vi "Autonomous Independent.vi"   [LabVIEW 2015]
doc: "This VI is called when autonomous begins, and will automatically be terminated when autonomous ends. You can carry out timed or sensor driven robot movement independently without needing to return to the caller."
uses:
  <vilib>/Rock Robotics/WPI/Utilities/WPI_GetSetVariantRefNum.vi
  <vilib>/Rock Robotics/Network Tables/NT Read String.vi
  <vilib>/Rock Robotics/Network Tables/NT Write Numeric Array.vi
  <vilib>/Rock Robotics/WPI/RobotDrive/WPI_RobotDriveArcadeDrive_Standard(NoSaturation).vi
  Robot Global Data.vi
panel:
  # "Be sure to right-click and choose Data Operations>>Make Current Value default if you want to save the array values with the VI"
types:
  T1 = typedef "WPI_JoystickDevRef.ctl" = cluster{"Device":T2}
  T2 = typedef "WPI_JoystickDeviceEnum.ctl" = enum16{"USB 0", "USB 1", "USB 2", "USB 3", "USB 4", "USB 5"}
  T3 = typedef "WPI_RobotDriveDevRef.ctl" = cluster{"DevStatus":errorcluster, "Motors[]":T4[], "Square Inputs":bool, "Max Output":dbl}
  T4 = typedef "WPI_MotorControlDeviceRef.ctl" = cluster{"DeviceStatus":errorcluster, "Type":T5, "PWM":cluster{"PWM Channel":T6, "DeadBand":T7}, "CAN":cluster{"Device Number":u8, "Control Mode":T8, "Semaphore":T9, "Max Vout":dbl, "TalonSRX Control Mode":T10}, "Invert":bool}
  T5 = typedef "WPI_MotorControlType.ctl" = enum16{"PWM", "CAN", "CANTalonSRX"}
  T6 = typedef "FPGA_DIOPWMChannel.ctl" = enum8{"PWM 0", "PWM 1", "PWM 2", "PWM 3", "PWM 4", "PWM 5", "PWM 6", "PWM 7", "PWM 8", "PWM 9", "PWM MXP 0", "PWM MXP 1", "PWM MXP 2", "PWM MXP 3", "PWM MXP 4", "PWM MXP 5", "PWM MXP 6", "PWM MXP 7", "PWM MXP 8", "PWM MXP 9", "Invalid"}
  T7 = typedef "WPI_PWMDeadband.ctl" = cluster{"Name":string, "maxPositivePwm":i32, "minPositivePwm":i32, "centerPwm":i32, "maxNegativePwm":i32, "minNegativePwm":i32, "angularRange":u16}
  T8 = typedef "WPI_CANJaguar_ControlMode.ctl" = enum8{"Percent VBus", "Current", "Speed", "Position", "Voltage"}
  T9 = typedef "Semaphore RefNum" = refnum<k1>
  T10 = typedef "WPI_CANTalonSRX_APIControlMode.ctl" = enum8{"Percent VBus", "Speed", "Position", "Slave", "Unchanged / Invalid", "Voltage Compensation", "Current", "Motion Profile"}
  T11 = typedef "WPI_AnalogChannelDevRef.ctl" = cluster{"DevStatus":errorcluster, "Analog Channel":T12}
  T12 = typedef "FPGA_AIChannel.ctl" = enum8{"AI 0", "AI 1", "AI 2", "AI 3", "AI MXP 0", "AI MXP 1", "AI MXP 2", "AI MXP 3", "Invalid"}
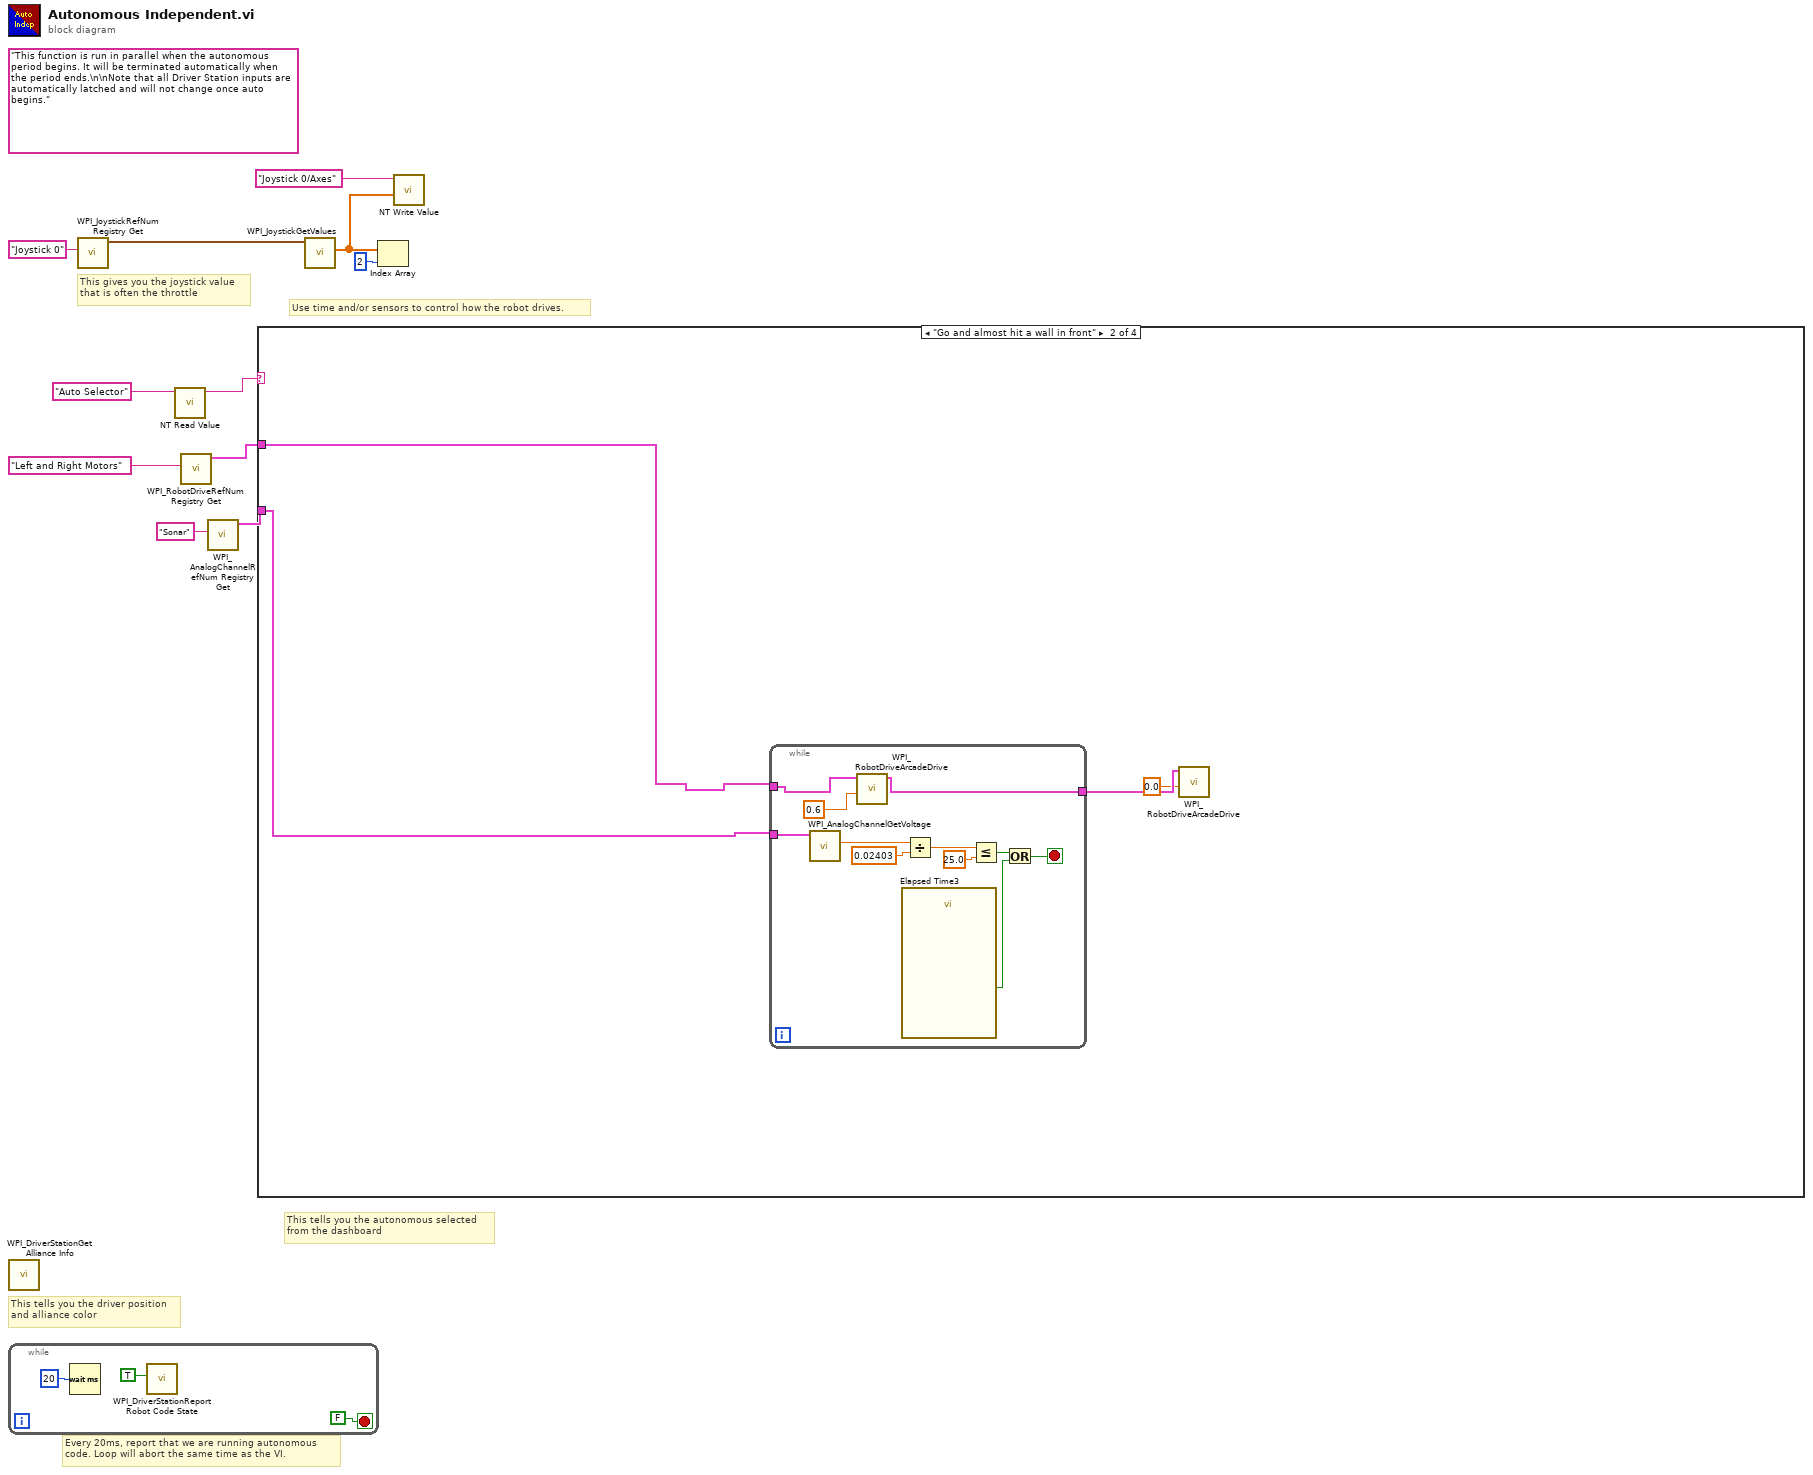
[diagram p0: block diagram]
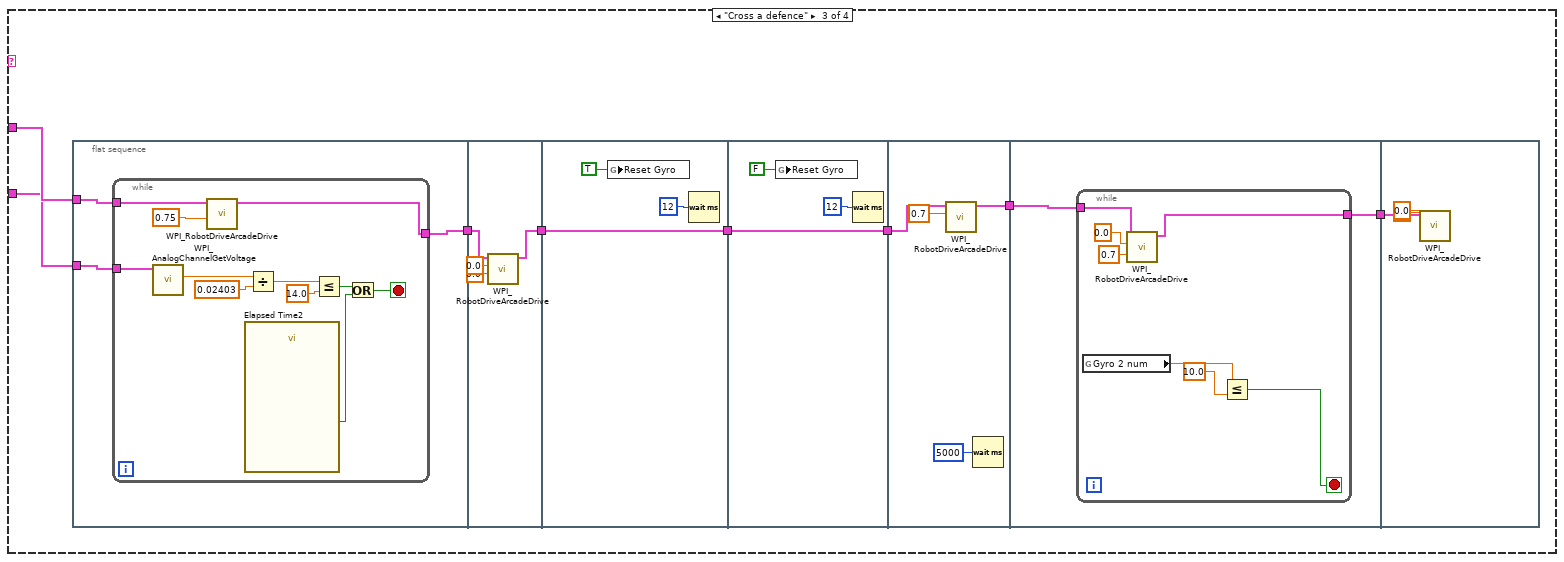
[diagram p3: hidden frame]
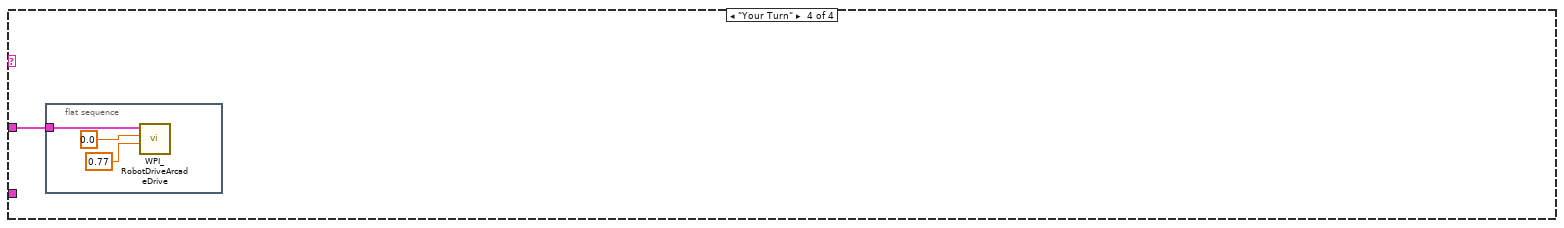
[diagram p4: hidden frame]
diagram:
  (unwired) "This function is run in parallel when the autonomous period begins. It will be terminated automatically when the period ends.\n\nNote that all Driver Station inputs are automatically latched and will not change once auto begins."
  # "This tells you the autonomous selected\nfrom the dashboard"
  # "Every 20ms, report that we are running autonomous\ncode. Loop will abort the same time as the VI."
  # "This gives you the joystick value\nthat is often the throttle"
  # "Use time and/or sensors to control how the robot drives."
  # "This tells you the driver position\nand alliance color"
  n1 = call <vilib>:"WPI_DriverStationGet Alliance Info.vi"() -> ()  [unwired: 12 out]
  n2 = while {
    stop <- FALSE stop-if-true
    n3 = Wait (ms)(milliseconds to wait=u32 20) -> ()  [unwired: 1 out]
    n4 = call <vilib>:"WPI_DriverStationReport Robot Code State.vi"("Autonomous"=TRUE) -> ()  [unwired: 10 in, 1 out]
  }
  n5 = call <vilib>:"WPI_JoystickRefNum Registry Get.vi"("refnum name"="Joystick 0") -> ("JoystickDevRef"=w10:T1)  [unwired: 1 in, 9 out]
  n6 = call-poly <vilib>:"NT Read Value.vi"("Name"="Auto Selector") -> ("String"=w7:string)  [unwired: 9 in, 1 out]
  n7 = call <vilib>:"WPI_RobotDriveRefNum Registry Get.vi"("refnum name"="Left and Right Motors") -> ("RobotDriveDevRef"=w3:T3)  [unwired: 9 in, 1 out]
  n8 = call <vilib>:"WPI_AnalogChannelRefNum Registry Get.vi"("refnum name"="Sonar") -> ("AIDeviceRef"=w1:T11)  [unwired: 9 in, 1 out]
  n9 = case shown="\"Go and almost hit a wall in front\"" w7 {
    tunnel: w1 -> [_ w18 w36 _]
    tunnel: w3 -> [_ w15 w37 w78]
    frame Default {
      # "You can put your main auto here, or you can right-click on the case and make any\nother frame be the default case."
      # "This is the frame that will execute if no selection is made, or if it is not recognized"
    }
    frame "Go and almost hit a wall in front" {
      n10 = while {
        tunnel: w18 -> [w28]
        tunnel: w15 -> [w20]
        tunnel: [w19] -> w17
        stop <- w23 stop-if-true
        n11 = call <vilib>:"WPI_AnalogChannelGetVoltage.vi"("AIDeviceRef"=w28) -> ("Voltage"=w27:dbl)  [unwired: 8 in, 2 out]
        n12 = call-poly <vilib>:"WPI_RobotDriveArcadeDrive.vi"("Y axis value"=0.6, "RobotDriveDevRef"=w20) -> ("RobotDriveDevRef"=w19:T3)  [unwired: 7 in, 2 out]
        n13 = call "Elapsed Time3"() -> ("Time has Elapsed"=w22:bool)  [unwired: 12 in, 7 out]
        n14 = Divide(x=w27, y=0.02403) -> (x/y=w25:dbl)
        n15 = Less Or Equal?(x=w25, y=25.0) -> (x <= y?=w24:bool)
        n16 = Or(x=w24, y=w22) -> (x .or. y?=w23:bool)
      }
      n17 = call-poly <vilib>:"WPI_RobotDriveArcadeDrive.vi"("Y axis value"=0.0, "RobotDriveDevRef"=w17) -> ()  [unwired: 7 in, 3 out]
    }
    frame "Cross a defence" {
      n18 = flat-sequence {
        tunnel: w37 -> [w40]
        tunnel: w36 -> [w39]
        tunnel: [w38] -> w31
        tunnel: w31 -> [w55]
        tunnel: [w54] -> w30
        tunnel: [w56] -> w34
        tunnel: w30 -> [w56]
        tunnel: [w59] -> w35
        tunnel: w34 -> [w59]
        tunnel: w35 -> [w65]
        tunnel: [w62] -> w33
        tunnel: w33 -> [w67]
        tunnel: [w66] -> w32
        tunnel: w32 -> [w77]
        frame #0 {
          n19 = while {
            tunnel: w39 -> [w49]
            tunnel: w40 -> [w51]
            tunnel: [w41] -> w38
            stop <- w43 stop-if-true
            n20 = call <vilib>:"WPI_AnalogChannelGetVoltage.vi"("AIDeviceRef"=w49) -> ("Voltage"=w48:dbl)  [unwired: 8 in, 2 out]
            n21 = call-poly <vilib>:"WPI_RobotDriveArcadeDrive.vi"("Y axis value"=0.75 ("X axis value"), "RobotDriveDevRef"=w51) -> ("RobotDriveDevRef"=w41:T3)  [unwired: 7 in, 2 out]
            n22 = call "Elapsed Time2"() -> ("Time has Elapsed"=w42:bool)  [unwired: 12 in, 7 out]
            n23 = Divide(x=w48, y=0.02403) -> (x/y=w46:dbl)
            n24 = Less Or Equal?(x=w46, y=14.0) -> (x <= y?=w44:bool)
            n25 = Or(x=w44, y=w42) -> (x .or. y?=w43:bool)
          }
        }
        frame #1 {
          n26 = call-poly <vilib>:"WPI_RobotDriveArcadeDrive.vi"("Y axis value"=0.0, "X axis value"=0.0, "RobotDriveDevRef"=w55) -> ("RobotDriveDevRef"=w54:T3)  [unwired: 6 in, 2 out]
        }
        frame #2 {
          n27 = global write "Robot Global Data.vi" "Reset Gyro"(TRUE) -> ()
          n28 = Wait (ms)(milliseconds to wait=u32 12) -> ()  [unwired: 1 out]
        }
        frame #3 {
          n29 = global write "Robot Global Data.vi" "Reset Gyro"(FALSE ("Reset Gyro")) -> ()
          n30 = Wait (ms)(milliseconds to wait=u32 12) -> ()  [unwired: 1 out]
        }
        frame #4 {
          n31 = call-poly <vilib>:"WPI_RobotDriveArcadeDrive.vi"("X axis value"=0.7, "RobotDriveDevRef"=w65) -> ("RobotDriveDevRef"=w62:T3)  [unwired: 7 in, 2 out]
          n32 = Wait (ms)(milliseconds to wait=u32 5000) -> ()  [unwired: 1 out]
        }
        frame #5 {
          n33 = while {
            tunnel: w67 -> [w70]
            tunnel: [w68] -> w66
            stop <- w69 stop-if-true
            n34 = global read "Robot Global Data.vi" "Gyro 2 num"() -> (w74:dbl)
            n35 = call-poly <vilib>:"WPI_RobotDriveArcadeDrive.vi"("Y axis value"=0.7, "X axis value"=0.0, "RobotDriveDevRef"=w70) -> ("RobotDriveDevRef"=w68:T3)  [unwired: 6 in, 2 out]
            n36 = Less Or Equal?(x=w74, y=10.0) -> (x <= y?=w69:bool)
          }
        }
        frame #6 {
          n37 = call-poly <vilib>:"WPI_RobotDriveArcadeDrive.vi"("Y axis value"=0.0, "X axis value"=0.0, "RobotDriveDevRef"=w77) -> ()  [unwired: 6 in, 3 out]
        }
      }
    }
    frame "Your Turn" {
      n38 = flat-sequence {
        tunnel: w78 -> [w79]
        frame #0 {
          n39 = call-poly <vilib>:"WPI_RobotDriveArcadeDrive.vi"("Y axis value"=0.77 ("RightSpeed"), "X axis value"=0.0 ("LeftSpeed"), "RobotDriveDevRef"=w79) -> ()  [unwired: 6 in, 3 out]
        }
      }
    }
  }
  n40 = call <vilib>:"WPI_JoystickGetValues.vi"("JoystickDevRef"=w10) -> ("Axes"=w6:dbl[])  [unwired: 6 in, 4 out]
  n41 = Index Array(array=w6, index=2) -> ()  [unwired: 1 out]
  n42 = call-poly <vilib>:"NT Write Value.vi"("Numeric Array"=w6, "Name"="Joystick 0/Axes") -> ()  [unwired: 9 in, 1 out]
